vi "USBRelay.vi"(11 "继电器开关":bool) -> ()   [LabVIEW 2014]
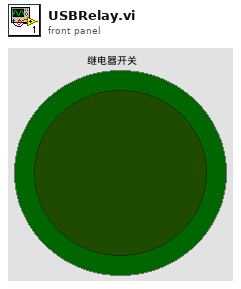
[diagram p1: front panel]
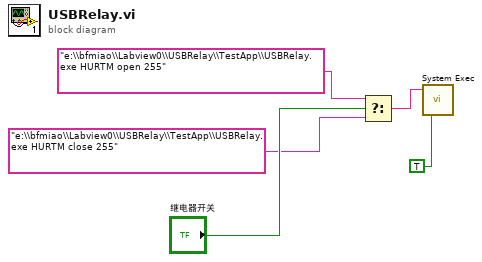
[diagram p0: block diagram]
diagram:
  n1 = Select(t="e:\\bfmiao\\Labview0\\USBRelay\\TestApp\\USBRelay.exe HURTM open 255", s="继电器开关", f="e:\\bfmiao\\Labview0\\USBRelay\\TestApp\\USBRelay.exe HURTM close 255") -> (s? t:f=w1:string)
  n2 = call <vilib>:"System Exec.vi"("run minimized? (F)"=TRUE, "command line"=w1) -> ()  [unwired: 6 in, 4 out]
